vi "Build Binary Stream From G Object.vi"(0 "TwinCAT ADS in":refnum<class "TwinCAT ADS.lvclass">, 5 "Value":variant, 7 "Type Name":string, 9 ".NET Ads Binary Writer":refnum<k24>, 11 "error in (no error)":errorcluster) -> (4 "TwinCAT ADS out":refnum<class "TwinCAT ADS.lvclass">, 15 "error out":errorcluster)   [LabVIEW 2018, in "TwinCAT ADS.lvclass"]
uses:
  TwinCAT ADS.lvclass
  TwinCAT.Ads
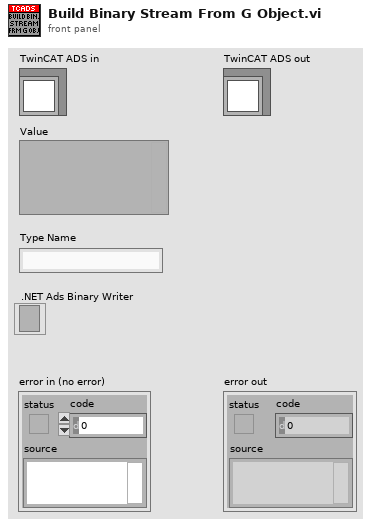
[diagram p1: front panel]
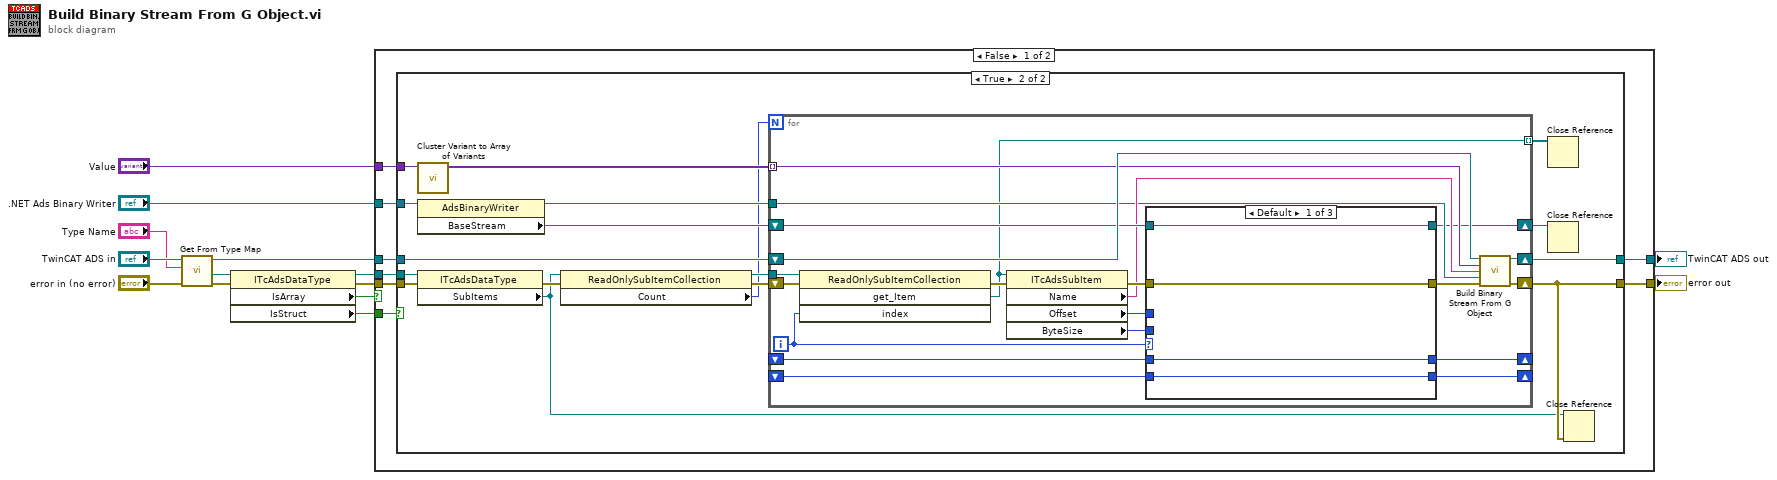
[diagram p0: block diagram]
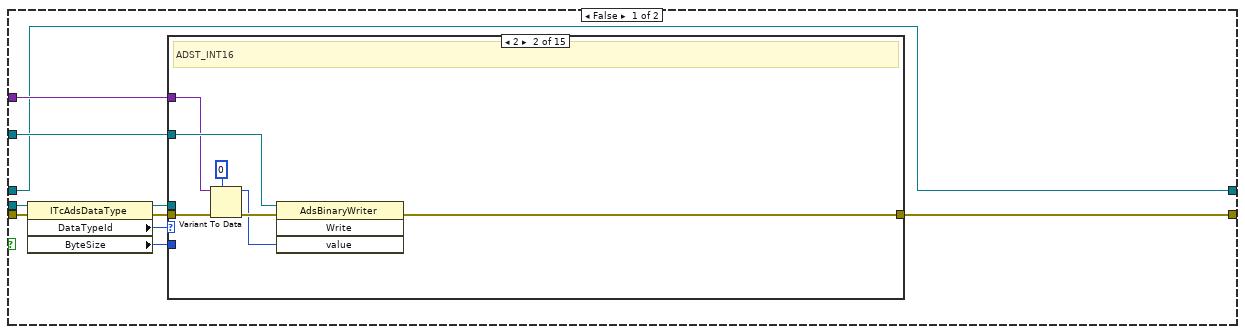
[diagram p2: hidden frame]
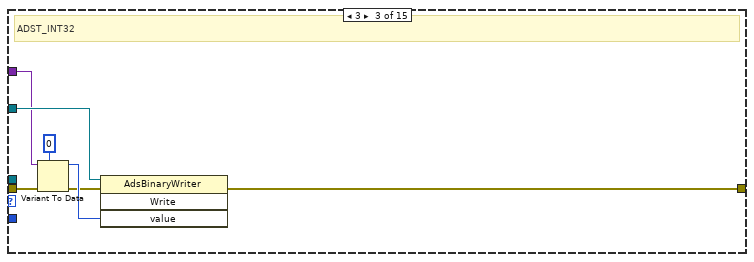
[diagram p4: hidden frame]
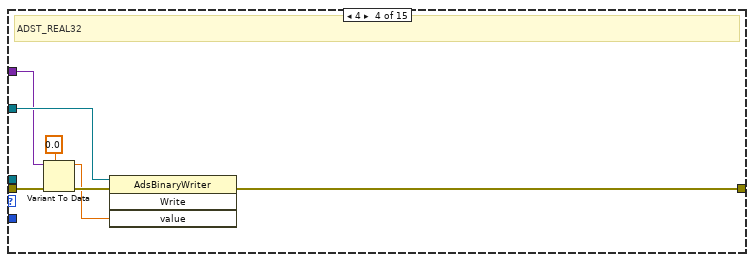
[diagram p5: hidden frame]
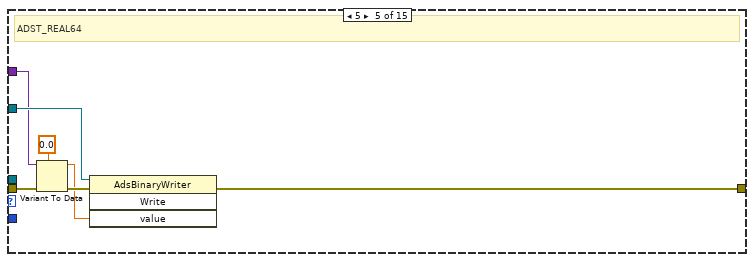
[diagram p6: hidden frame]
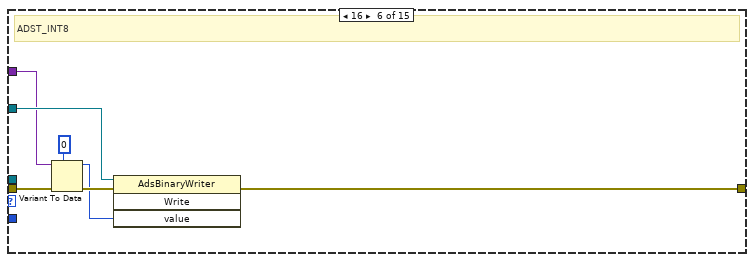
[diagram p7: hidden frame]
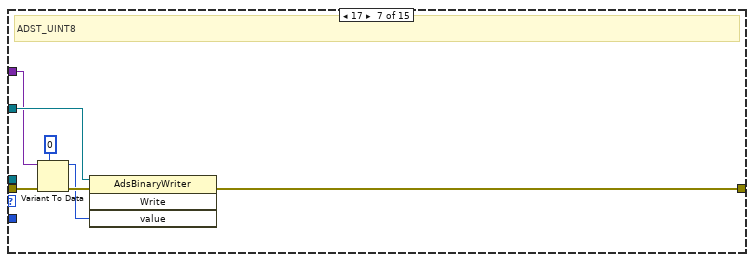
[diagram p8: hidden frame]
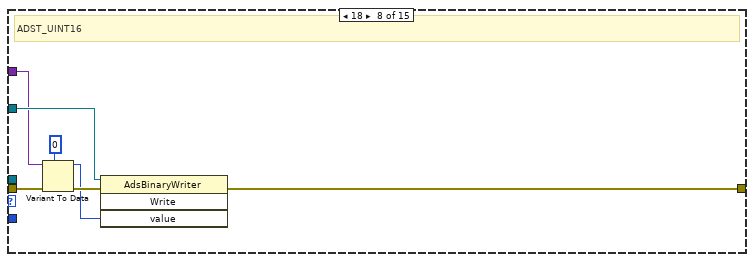
[diagram p9: hidden frame]
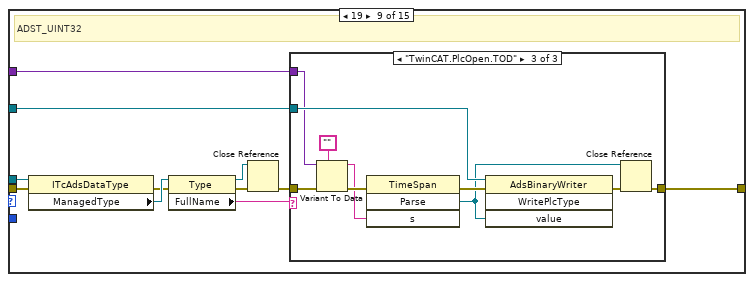
[diagram p10: hidden frame]
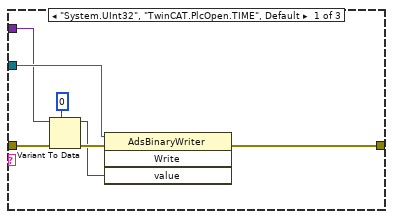
[diagram p11: hidden frame]
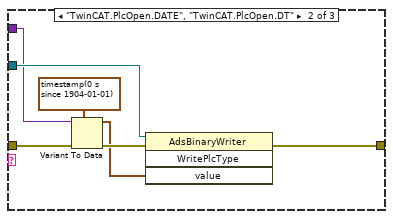
[diagram p12: hidden frame]
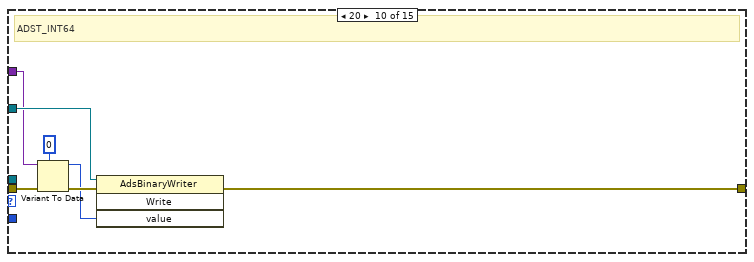
[diagram p13: hidden frame]
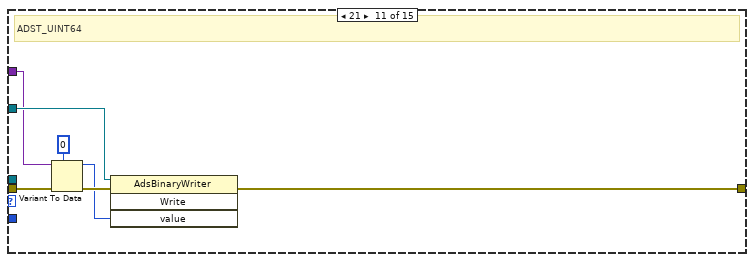
[diagram p14: hidden frame]
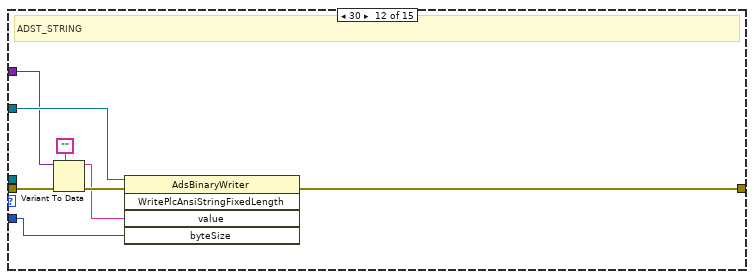
[diagram p15: hidden frame]
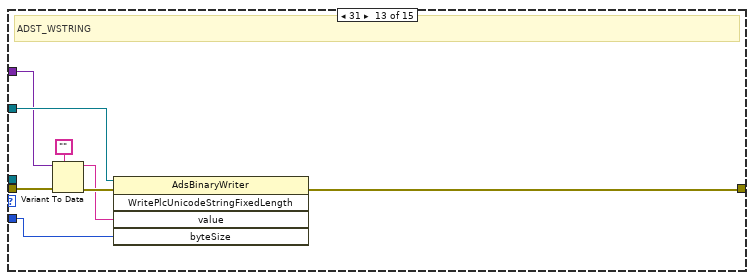
[diagram p16: hidden frame]
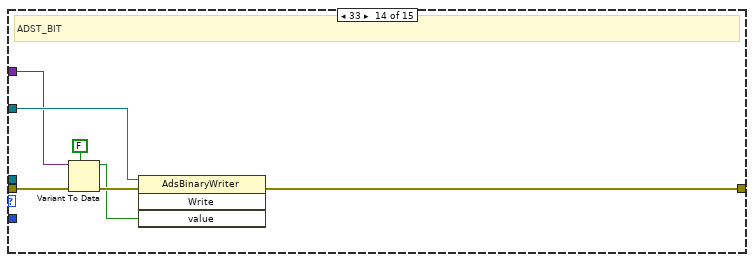
[diagram p17: hidden frame]
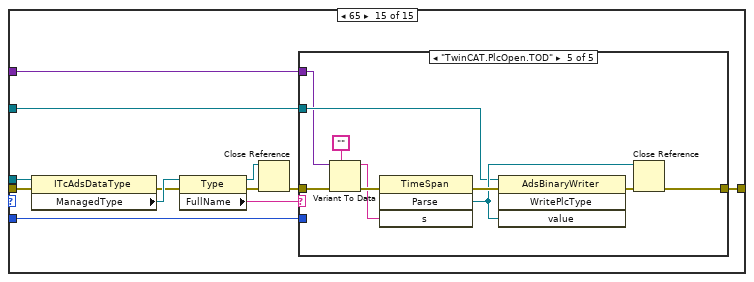
[diagram p18: hidden frame]
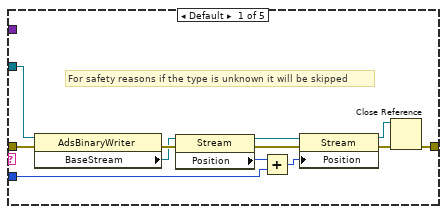
[diagram p19: hidden frame]
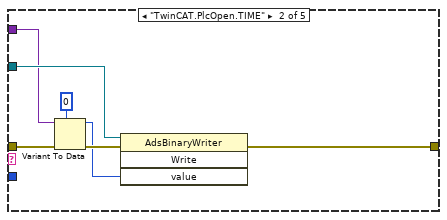
[diagram p20: hidden frame]
diagram:
  n1 = call "Get From Type Map.vi"("error in (no error)"="error in (no error)", "Type Name"="Type Name", "TwinCAT ADS in"="TwinCAT ADS in") -> ("error out"=w11:errorcluster, ".NET AdsDataType"=w10:refnum<k24>, "TwinCAT ADS out"=w7:refnum<class "TwinCAT ADS.lvclass">)  [unwired: 6 in]
  n2 = property class="ITcAdsDataType"(reference=w10, error in=w11) -> (reference out=w5:refnum<k24>, error out=w6:errorcluster, "IsArray"=w9:bool, "IsStruct"=w8:bool)
  n3 = case shown="False" w9 {
    tunnel: w8 -> [w22 _]
    tunnel: w7 -> [w19 w275]
    tunnel: w6 -> [w21 w284]
    tunnel: w5 -> [w20 w283]
    tunnel: [w17 w270] -> w4
    tunnel: [w18 w271] -> w3
    tunnel: ".NET Ads Binary Writer" -> [w16 w272]
    tunnel: "Value" -> [w15 w278]
    frame False {
      n4 = case shown="True" w22 {
        tunnel: w21 -> [w32 w223]
        tunnel: w20 -> [w31 w222]
        tunnel: w19 -> [w23 w221]
        tunnel: [w24 w211] -> w18
        tunnel: [w23 w214] -> w17
        tunnel: w16 -> [w27 w226]
        tunnel: w15 -> [w26 w225]
        frame False {
          n5 = property class="ITcAdsDataType"(reference=w31, error in=w32) -> (reference out=w25:refnum<k24>, error out=w30:errorcluster, "DataTypeId"=w29:i32, "ByteSize"=w28:i32)
          n6 = case shown="2" w29 {
            tunnel: w30 -> [w33 w38 w42 w51 w59 w65 w73 w80 w86 w124 w128 w136 w144 w152 w159]
            tunnel: w28 -> [_ _ _ _ _ _ _ _ _ _ _ w137 w142 _ w156]
            tunnel: w27 -> [_ w40 w47 w54 w61 w68 w75 w82 w90 w120 w127 w139 w143 w154 w161]
            tunnel: [w33 w39 w46 w53 w60 w67 w74 w81 w93 w118 w125 w138 w140 w153 w160] -> w24
            tunnel: w25 -> [_ _ _ _ _ _ _ _ w85 _ _ _ _ _ w158]
            tunnel: w26 -> [_ w34 w45 w49 w55 w62 w71 w79 w83 w119 w126 w133 w141 w148 w155]
            frame 0, Default {
              # "ADST_VOID"
            }
            frame 2 {
              # "ADST_INT16"
              n7 = Variant To Data(error in=w38, type=i16 0 ("value"), Variant=w34) -> (data=w35:i16, error out=w37:errorcluster)
              n8 = invoke class="AdsBinaryWriter" method="Write"(reference=w40, error in=w37, "value"=w35) -> (error out=w39:errorcluster)  [unwired: 1 in, 3 out]
            }
            frame 3 {
              # "ADST_INT32"
              n9 = Variant To Data(error in=w42, type=0 ("value"), Variant=w45) -> (data=w43:i32, error out=w41:errorcluster)
              n10 = invoke class="AdsBinaryWriter" method="Write"(reference=w47, error in=w41, "value"=w43) -> (error out=w46:errorcluster)  [unwired: 1 in, 3 out]
            }
            frame 4 {
              # "ADST_REAL32"
              n11 = Variant To Data(error in=w51, type=sgl 0.0 ("value"), Variant=w49) -> (data=w48:sgl, error out=w50:errorcluster)
              n12 = invoke class="AdsBinaryWriter" method="Write"(reference=w54, error in=w50, "value"=w48) -> (error out=w53:errorcluster)  [unwired: 1 in, 3 out]
            }
            frame 5 {
              # "ADST_REAL64"
              n13 = Variant To Data(error in=w59, type=0.0 ("value"), Variant=w55) -> (data=w57:dbl, error out=w58:errorcluster)
              n14 = invoke class="AdsBinaryWriter" method="Write"(reference=w61, error in=w58, "value"=w57) -> (error out=w60:errorcluster)  [unwired: 1 in, 3 out]
            }
            frame 16 {
              # "ADST_INT8"
              n15 = Variant To Data(error in=w65, type=i8 0 ("value"), Variant=w62) -> (data=w63:i8, error out=w64:errorcluster)
              n16 = invoke class="AdsBinaryWriter" method="Write"(reference=w68, error in=w64, "value"=w63) -> (error out=w67:errorcluster)  [unwired: 1 in, 3 out]
            }
            frame 17 {
              # "ADST_UINT8"
              n17 = Variant To Data(error in=w73, type=u8 0 ("value"), Variant=w71) -> (data=w69:u8, error out=w72:errorcluster)
              n18 = invoke class="AdsBinaryWriter" method="Write"(reference=w75, error in=w72, "value"=w69) -> (error out=w74:errorcluster)  [unwired: 1 in, 3 out]
            }
            frame 18 {
              # "ADST_UINT16"
              n19 = Variant To Data(error in=w80, type=u16 0 ("value"), Variant=w79) -> (data=w76:u16, error out=w77:errorcluster)
              n20 = invoke class="AdsBinaryWriter" method="Write"(reference=w82, error in=w77, "value"=w76) -> (error out=w81:errorcluster)  [unwired: 1 in, 3 out]
            }
            frame 19 {
              # "ADST_UINT32"
              n21 = property class="ITcAdsDataType"(reference=w85, error in=w86) -> (error out=w84:errorcluster, "ManagedType"=w92:refnum<k24>)  [unwired: 1 out]
              n22 = property class="Type"(reference=w92, error in=w84) -> (reference out=w87:refnum<k24>, error out=w89:errorcluster, "FullName"=w91:string)
              n23 = Close Reference(reference=w87, error in (no error)=w89) -> (error out=w88:errorcluster)
              n24 = case shown="\"TwinCAT.PlcOpen.TOD\"" w91 {
                tunnel: [w94 w101 w112] -> w93
                tunnel: w88 -> [w99 w106 w117]
                tunnel: w90 -> [w98 w103 w114]
                tunnel: w83 -> [w97 w102 w110]
                frame "System.UInt32", "TwinCAT.PlcOpen.TIME", Default {
                  n25 = Variant To Data(error in=w99, type=u32 0 ("value"), Variant=w97) -> (data=w95:u32, error out=w100:errorcluster)
                  n26 = invoke class="AdsBinaryWriter" method="Write"(reference=w98, error in=w100, "value"=w95) -> (error out=w94:errorcluster)  [unwired: 1 in, 3 out]
                }
                frame "TwinCAT.PlcOpen.DATE", "TwinCAT.PlcOpen.DT" {
                  n27 = Variant To Data(error in=w106, type=timestamp(0 s since 1904-01-01) ("value"), Variant=w102) -> (data=w104:timestamp, error out=w107:errorcluster)
                  n28 = invoke class="AdsBinaryWriter" method="WritePlcType"(reference=w103, error in=w107, "value"=w104) -> (error out=w101:errorcluster)  [unwired: 1 in, 3 out]
                }
                frame "TwinCAT.PlcOpen.TOD" {
                  n29 = Variant To Data(error in=w117, type="", Variant=w110) -> (data=w108:string, error out=w116:errorcluster)
                  n30 = invoke class="TimeSpan" method="Parse"(error in=w116, "s"=w108) -> (error out=w115:errorcluster, "Parse"=w111:refnum<k24>)  [unwired: 2 in, 2 out]
                  n31 = invoke class="AdsBinaryWriter" method="WritePlcType"(reference=w114, error in=w115, "value"=w111) -> (error out=w113:errorcluster)  [unwired: 1 in, 3 out]
                  n32 = Close Reference(reference=w111, error in (no error)=w113) -> (error out=w112:errorcluster)
                }
              }
            }
            frame 20 {
              # "ADST_INT64"
              n33 = Variant To Data(error in=w124, type=i64 0 ("value"), Variant=w119) -> (data=w121:i64, error out=w122:errorcluster)
              n34 = invoke class="AdsBinaryWriter" method="Write"(reference=w120, error in=w122, "value"=w121) -> (error out=w118:errorcluster)  [unwired: 1 in, 3 out]
            }
            frame 21 {
              # "ADST_UINT64"
              n35 = Variant To Data(error in=w128, type=u64 0 ("value"), Variant=w126) -> (data=w129:u64, error out=w130:errorcluster)
              n36 = invoke class="AdsBinaryWriter" method="Write"(reference=w127, error in=w130, "value"=w129) -> (error out=w125:errorcluster)  [unwired: 1 in, 3 out]
            }
            frame 30 {
              # "ADST_STRING"
              n37 = Variant To Data(error in=w136, type="", Variant=w133) -> (data=w132:string, error out=w134:errorcluster)
              n38 = invoke class="AdsBinaryWriter" method="WritePlcAnsiStringFixedLength"(reference=w139, error in=w134, "value"=w132, "byteSize"=w137) -> (error out=w138:errorcluster)  [unwired: 1 in, 4 out]
            }
            frame 31 {
              # "ADST_WSTRING"
              n39 = Variant To Data(error in=w144, type="", Variant=w141) -> (data=w145:string, error out=w146:errorcluster)
              n40 = invoke class="AdsBinaryWriter" method="WritePlcUnicodeStringFixedLength"(reference=w143, error in=w146, "value"=w145, "byteSize"=w142) -> (error out=w140:errorcluster)  [unwired: 1 in, 4 out]
            }
            frame 33 {
              # "ADST_BIT"
              n41 = Variant To Data(error in=w152, type=FALSE, Variant=w148) -> (data=w149:bool, error out=w151:errorcluster)
              n42 = invoke class="AdsBinaryWriter" method="Write"(reference=w154, error in=w151, "value"=w149) -> (error out=w153:errorcluster)  [unwired: 1 in, 3 out]
            }
            frame 65 {
              n43 = property class="ITcAdsDataType"(reference=w158, error in=w159) -> (error out=w157:errorcluster, "ManagedType"=w166:refnum<k24>)  [unwired: 1 out]
              n44 = property class="Type"(reference=w166, error in=w157) -> (reference out=w164:refnum<k24>, error out=w165:errorcluster, "FullName"=w163:string)
              n45 = Close Reference(reference=w164, error in (no error)=w165) -> (error out=w162:errorcluster)
              n46 = case shown="\"TwinCAT.PlcOpen.TOD\"" w163 {
                tunnel: w162 -> [w177 w183 w190 w196 w203]
                tunnel: w161 -> [w178 w185 w192 w195 w202]
                tunnel: [w174 w184 w191 w193 w201] -> w160
                tunnel: w156 -> [w168 _ _ _ _]
                tunnel: w155 -> [_ w182 w189 w194 w200]
                frame Default {
                  # "For safety reasons if the type is unknown it will be skipped"
                  n47 = property class="AdsBinaryWriter"(reference=w178, error in=w177) -> (error out=w176:errorcluster, "BaseStream"=w175:refnum<k24>)  [unwired: 1 out]
                  n48 = property class="Stream"(reference=w175, error in=w176) -> (reference out=w170:refnum<k24>, error out=w171:errorcluster, "Position"=w169:i64)
                  n49 = Add(x=w169, y=w168) -> (x+y=w167:i64)
                  n50 = property class="Stream"(reference=w170, error in=w171, "Position"=w167) -> (reference out=w172:refnum<k24>, error out=w173:errorcluster)
                  n51 = Close Reference(reference=w172, error in (no error)=w173) -> (error out=w174:errorcluster)
                }
                frame "TwinCAT.PlcOpen.TIME" {
                  n52 = Variant To Data(error in=w183, type=u32 0, Variant=w182) -> (data=w179:u32, error out=w181:errorcluster)
                  n53 = invoke class="AdsBinaryWriter" method="Write"(reference=w185, error in=w181, "value"=w179) -> (error out=w184:errorcluster)  [unwired: 1 in, 3 out]
                }
                frame "TwinCAT.PlcOpen.LTIME" {
                  n54 = Variant To Data(error in=w190, type=u64 0, Variant=w189) -> (data=w186:u64, error out=w188:errorcluster)
                  n55 = invoke class="AdsBinaryWriter" method="Write"(reference=w192, error in=w188, "value"=w186) -> (error out=w191:errorcluster)  [unwired: 1 in, 3 out]
                }
                frame "TwinCAT.PlcOpen.DATE", "TwinCAT.PlcOpen.DT" {
                  n56 = Variant To Data(error in=w196, type=timestamp(0 s since 1904-01-01) ("value"), Variant=w194) -> (data=w197:timestamp, error out=w199:errorcluster)
                  n57 = invoke class="AdsBinaryWriter" method="WritePlcType"(reference=w195, error in=w199, "value"=w197) -> (error out=w193:errorcluster)  [unwired: 1 in, 3 out]
                }
                frame "TwinCAT.PlcOpen.TOD" {
                  n58 = Variant To Data(error in=w203, type="", Variant=w200) -> (data=w204:string, error out=w209:errorcluster)
                  n59 = invoke class="TimeSpan" method="Parse"(error in=w209, "s"=w204) -> (error out=w208:errorcluster, "Parse"=w206:refnum<k24>)  [unwired: 2 in, 2 out]
                  n60 = invoke class="AdsBinaryWriter" method="WritePlcType"(reference=w202, error in=w208, "value"=w206) -> (error out=w207:errorcluster)  [unwired: 1 in, 3 out]
                  n61 = Close Reference(reference=w206, error in (no error)=w207) -> (error out=w201:errorcluster)
                }
              }
            }
          }
        }
        frame True {
          n62 = call "Cluster Variant to Array of Variants.vi"("Cluster Variant"=w225) -> ("[Variant]"=w218:variant[])  [unwired: 9 in, 1 out]
          n63 = property class="AdsBinaryWriter"(reference=w226) -> (reference out=w219:refnum<k24>, "BaseStream"=w220:refnum<k24>)  [unwired: 1 in, 1 out]
          n64 = property class="ITcAdsDataType"(reference=w222, error in=w223) -> (error out=w224:errorcluster, "SubItems"=w210:refnum<k24>)  [unwired: 1 out]
          n65 = property class="ReadOnlySubItemCollection"(reference=w210, error in=w224) -> (reference out=w216:refnum<k24>, error out=w217:errorcluster, "Count"=w215:i32)
          n66 = for {
            N: w215 -> [_]
            shift-right: [w232] -> w214
            shift-left: w221 -> [w247]
            shift-right: [w228] -> w212
            shift-left: w220 -> [w239]
            tunnel: w219 -> [w229]
            tunnel: w218 -> [w231] mode=indexing
            shift-right: [w233] -> w211
            shift-left: w217 -> [w246]
            tunnel: w216 -> [w245]
            shift-right: [w238] -> _
            shift-left: _ -> [w237]
            shift-right: [w236] -> _
            shift-left: _ -> [w235]
            tunnel: [w227] -> w213 mode=indexing
            i -> [w243]
            n67 = invoke class="ReadOnlySubItemCollection" method="get_Item"(reference=w245, error in=w246, "index"=w243) -> (error out=w244:errorcluster, "get_Item"=w227:refnum<k24>)  [unwired: 1 in, 2 out]
            n68 = property class="ITcAdsSubItem"(reference=w227, error in=w244) -> (error out=w240:errorcluster, "Name"=w230:string, "Offset"=w241:i32, "ByteSize"=w242:i32)  [unwired: 1 out]
            n69 = case shown="Default" w243 {
              tunnel: w242 -> [_ w254 w260]
              tunnel: w241 -> [_ w253 w259]
              tunnel: w240 -> [w251 w255 w263]
              tunnel: [w251 w255 w256] -> w234
              tunnel: w239 -> [w248 w252 w262]
              tunnel: [w249 w254 w260] -> w236
              tunnel: [w250 w253 w259] -> w238
              tunnel: w237 -> [w250 _ w258]
              tunnel: w235 -> [w249 _ w257]
              tunnel: [w248 w252 w261] -> w228
              frame Default {
              }
              frame 0 {
              }
              frame 1.. {
                n70 = property class="Stream"(reference=w262, error in=w263) -> (reference out=w269:refnum<k24>, error out=w267:errorcluster, "Position"=w268:i64)
                n71 = Add(x=w258, y=w257) -> (x+y=w265:i32)
                n72 = Subtract(x=w259, y=w265) -> (x-y=w264:i32)
                n73 = Add(x=w268, y=w264) -> (x+y=w266:i64)
                n74 = property class="Stream"(reference=w269, error in=w267, "Position"=w266) -> (reference out=w261:refnum<k24>, error out=w256:errorcluster)
              }
            }
            n75 = call "Build Binary Stream From G Object.vi"("TwinCAT ADS in"=w247, "Value"=w231, "Type Name"=w230, ".NET Ads Binary Writer"=w229, "error in (no error)"=w234) -> ("TwinCAT ADS out"=w232:refnum<class "TwinCAT ADS.lvclass">, "error out"=w233:errorcluster)  [unwired: 9 in]
          }
          n76 = Close Reference(reference=w213) -> ()  [unwired: 1 in, 1 out]
          n77 = Close Reference(reference=w212) -> ()  [unwired: 1 in, 1 out]
          n78 = Close Reference(reference=w210, error in (no error)=w211) -> ()  [unwired: 1 out]
        }
      }
    }
    frame True {
      n79 = property class="ITcAdsDataType"(reference=w283, error in=w284) -> (error out=w282:errorcluster, "Dimensions"=w281:refnum<k24>, "BaseType"=w286:refnum<k24>)  [unwired: 1 out]
      n80 = call "Array Variant to Array of Variants.vi"("Arrray Variant"=w278) -> ("[Variant]"=w273:variant[])  [unwired: 9 in, 1 out]
      n81 = property class="ReadOnlyDimensionCollection"(reference=w281, error in=w282) -> (reference out=w279:refnum<k24>, error out=w280:errorcluster, "ElementCount"=w277:i32)
      n82 = property class="ITcAdsDataType"(reference=w286) -> (reference out=w285:refnum<k24>, "Name"=w276:string)  [unwired: 1 in, 1 out]
      n83 = Close Reference(reference=w285) -> ()  [unwired: 1 in, 1 out]
      n84 = Close Reference(reference=w279, error in (no error)=w280) -> (error out=w274:errorcluster)
      n85 = for {
        N: w277 -> [_]
        tunnel: w276 -> [w288]
        shift-right: [w291] -> w270
        shift-left: w275 -> [w293]
        shift-right: [w287] -> w271
        shift-left: w274 -> [w292]
        tunnel: w273 -> [w290] mode=indexing
        tunnel: w272 -> [w289]
        n86 = call "Build Binary Stream From G Object.vi"("TwinCAT ADS in"=w293, "Value"=w290, "Type Name"=w288, ".NET Ads Binary Writer"=w289, "error in (no error)"=w292) -> ("TwinCAT ADS out"=w291:refnum<class "TwinCAT ADS.lvclass">, "error out"=w287:errorcluster)  [unwired: 9 in]
      }
    }
  }
  "error out" <- w3
  "TwinCAT ADS out" <- w4
